vi "kalman.vi"() -> ()   [LabVIEW 2019]
uses:
  <vilib>/Utility/inputDevices.llb/mouseAcquire.vi
  labwindows/kalman.dll
panel:
  in  "noise":sgl
  in  "milliseconds to wait":u32
  out "actual":sgl[](array[numeric])
  out "cursor_pos":sgl[](array[numeric])
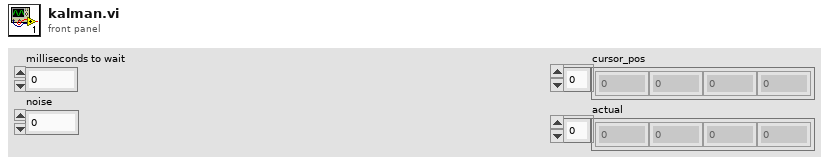
[diagram p1: front panel]
types:
  T1 = cluster{"Horizontal":i32, "Vertical":i32, "Scrolling":i32}
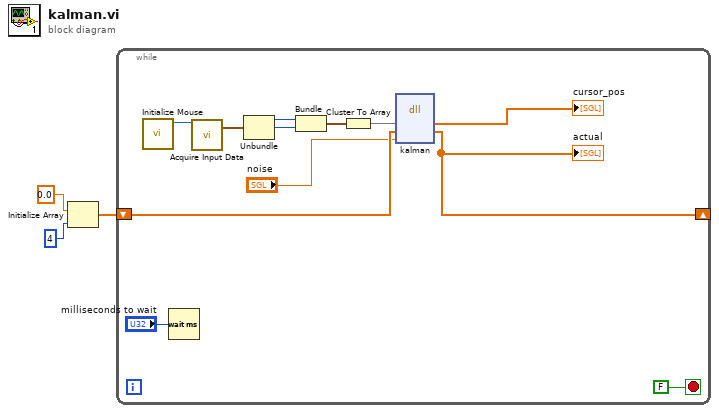
[diagram p0: block diagram]
diagram:
  n1 = Initialize Array(0.0 ("element"), 4 ("dimension size")) -> (w1:dbl[])
  n2 = while {
    shift-right: [w8] -> _
    shift-left: w1 -> [w9]
    stop <- FALSE stop-if-true
    n3 = call <vilib>:"Initialize Mouse.vi"() -> ("device ID"=w15:refnum<k1>)  [unwired: 10 in, 1 out]
    n4 = Wait (ms)(milliseconds to wait="milliseconds to wait") -> ()  [unwired: 1 out]
    n5 = call-poly <vilib>:"Acquire Input Data.vi"("device ID"=w15) -> ("axis info"=w14:T1)  [unwired: 15 in, 3 out]
    n6 = Unbundle(w14) -> ("Horizontal"=w13:i32, "Vertical"=w12:i32)  [unwired: 1 out]
    n7 = Bundle("Horizontal"=w13, "Vertical"=w12) -> (w11:cluster{"Horizontal":i32, "Vertical":i32})  [unwired: 1 in]
    n8 = Cluster To Array(cluster=w11) -> (array=w10:i32[])
    n9 = dll-call lib="C:/Users/aldemir/Desktop/mouse-tracker/labwindows/kalman.dll" fn="kalman"("cursor_pos"=w10, "actual"=w9, "noise"="noise") -> ("cursor_pos"=→"cursor_pos":sgl[], "actual"=w8:sgl[])  [unwired: 5 in, 2 out]
    "actual" <- w8
  }
